vi "mod_Phase Unwrap (Continuous).vi"(1 "Input Signal":dbl[](array[numeric]), 2 "Reset":bool) -> (0 "Phase Unwrapped":dbl[](array[numeric]))   [LabVIEW 2020, in "niAMT.lvlib"]
uses:
  <vilib>/addons/Modulation/niAMT.lvlib
  <vilib>/Analysis/NI_AALPro.lvlib
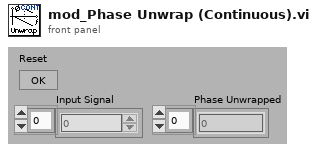
[diagram p1: front panel]
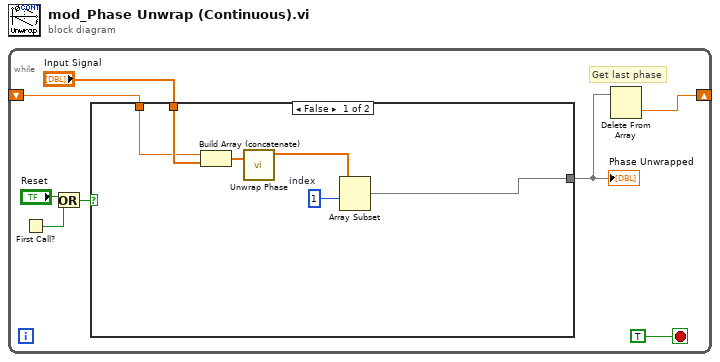
[diagram p0: block diagram]
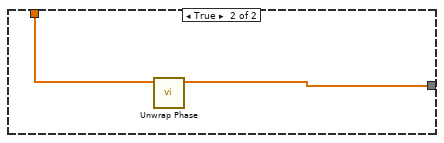
[diagram p2: hidden frame]
diagram:
  n1 = while {
    shift-right: [w6] -> _
    shift-left: _ -> [w5]
    stop <- TRUE stop-if-true
    # "Get last phase"
    n2 = First Call?() -> (First Call?: T/F=w2:bool)
    n3 = Or(x="Reset", y=w2) -> (x .or. y?=w1:bool)
    n4 = case shown="False" w1 {
      tunnel: "Input Signal" -> [w14 w16]
      tunnel: [w13 w15] -> w4
      tunnel: w5 -> [w12 _]
      frame False {
        w9 = 1  # index
        n5 = Build Array (concatenate)(w12, w14) -> (w11:dbl[])
        n6 = call <vilib>:"Unwrap Phase.vi"("Phase"=w11) -> ("Unwrapped Phase"=w10:dbl[])  [unwired: 1 in, 9 out]
        n7 = Array Subset(array=w10, index=w9) -> (w13:dbl[])  [unwired: 1 in]
      }
      frame True {
        n8 = call <vilib>:"Unwrap Phase.vi"("Phase"=w16) -> ("Unwrapped Phase"=w15:dbl[])  [unwired: 1 in, 9 out]
      }
    }
    "Phase Unwrapped" <- w4
    n9 = Delete From Array(array=w4) -> (deleted portion=w6:dbl)  [unwired: 2 in, 1 out]
  }
